vi "Format Message String.vi"(8 "error":errorcluster, 9 "ID":string, 10 "Data":string, 11 "Command":string) -> (3 "Message":string)   [LabVIEW 2019, in "RemoteControl.lvlib" / "RemoteControl.lvclass"]
uses:
  RemoteControl.lvclass
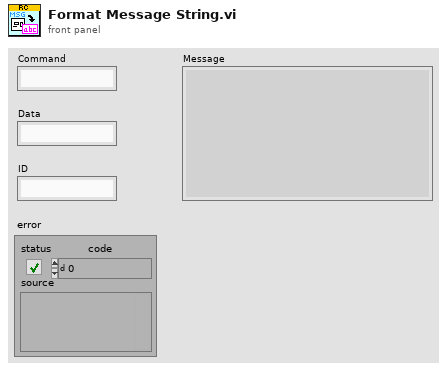
[diagram p1: front panel]
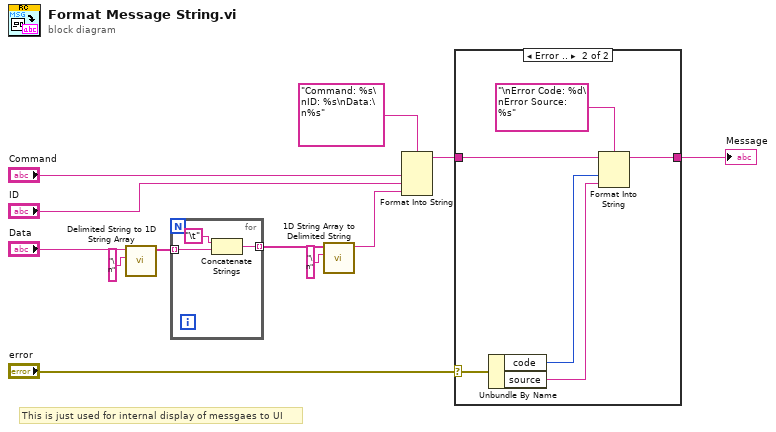
[diagram p0: block diagram]
diagram:
  # "This is just used for internal display of messgaes to UI"
  n1 = call <vilib>:"Delimited String to 1D String Array.vi"("delimiter"="\n", "delimited string"="Data") -> ("string array"=w11:string[])  [unwired: 9 in]
  n2 = for {
    tunnel: w11 -> [w15] mode=indexing
    tunnel: [w14] -> w10 mode=indexing
    n3 = Concatenate Strings("\t", w15) -> (w14:string)
  }
  n4 = call <vilib>:"1D String Array to Delimited String.vi"("delimiter"="\n", "string array"=w10) -> ("delimited string"=w6:string)  [unwired: 9 in]
  n5 = Format Into String(format string="Command: %s\nID: %s\nData:\n%s", "Command", "ID", w6) -> (resulting string=w1:string)  [unwired: 2 in, 1 out]
  n6 = case shown="Error .." "error" {
    selector: "error" -> [_ w22]
    tunnel: [w16 w20] -> w2
    tunnel: w1 -> [w16 w21]
    frame No Error {
    }
    frame Error {
      n7 = Unbundle By Name(w22) -> ("code"=w19:i32, "source"=w17:string)
      n8 = Format Into String(format string="\nError Code: %d\nError Source: %s", initial string=w21, w19, w17) -> (resulting string=w20:string)  [unwired: 1 in, 1 out]
    }
  }
  "Message" <- w2
